vi "Test TCP Socket.vi"() -> ()   [LabVIEW 2023]
panel:
  in  "Cluster":cluster{"1":dbl, "2":dbl}={"1"=4.0, "2"=12.1212}
  out "*(type *) &x":cluster{"1":dbl, "2":dbl}
  out "data string":string
  out "concatenated string":string
  out "data out":string
  out "error out":errorcluster
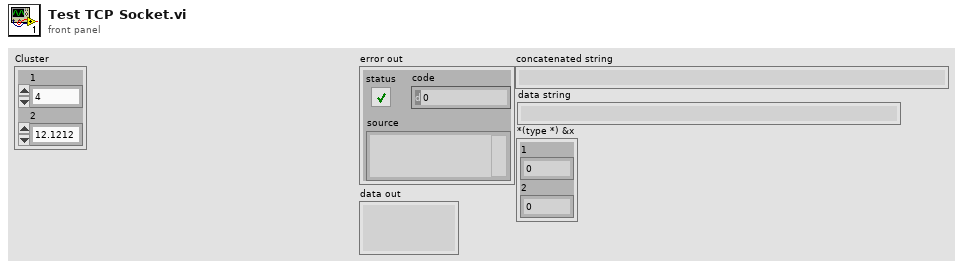
[diagram p1: front panel]
types:
  T1 = enum16{"Standard", "Buffered", "CRLF", "Immediate"}
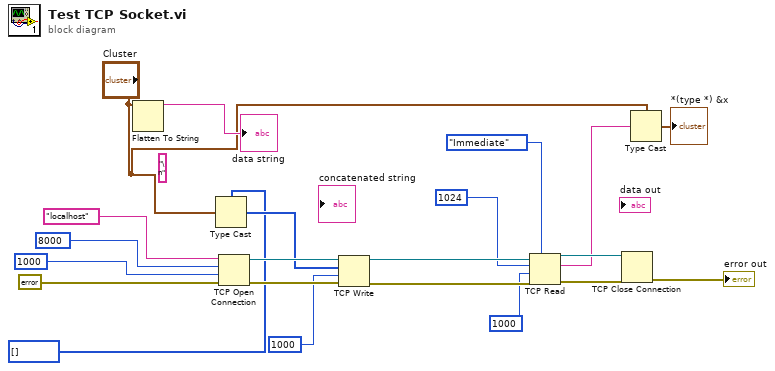
[diagram p0: block diagram]
diagram:
  (unwired) "\n"
  n1 = Flatten To String(anything="Cluster") -> (data string=→"data string":string)  [unwired: 3 in, 2 out]
  n2 = Type Cast(type=u8[] [], x="Cluster") -> (*(type *) &x=w5:u8[])
  n3 = TCP Open Connection(address="localhost", remote port or service name=u16 8000, timeout ms (60000)=1000, error in (no error)=errorcluster {"status"=FALSE, "code"=0, "source"=""}) -> (connection ID=w17:refnum<k5>, error out=w16:errorcluster)  [unwired: 1 in]
  n4 = TCP Write(connection ID=w17, data in=w5, error in (no error)=w16, 9:1000 ("timeout ms (25000)")) -> (connection ID out=w14:refnum<k5>, error out=w13:errorcluster)  [unwired: 1 out]
  n5 = TCP Read(connection ID=w14, bytes to read=1024, error in (no error)=w13, 7:T1."Immediate" ("mode (standard)"), 9:1000 ("timeout ms (25000)")) -> (connection ID out=w9:refnum<k5>, data out=w4:string, error out=w8:errorcluster)
  n6 = TCP Close Connection(connection ID=w9, error in (no error)=w8) -> (error out=→"error out":errorcluster)  [unwired: 1 in, 1 out]
  n7 = Type Cast(type="Cluster", x=w4) -> (*(type *) &x=→"*(type *) &x":cluster{"1":dbl, "2":dbl})
